vi "test Is OD Entry_3.vi"(11 "Test Case In":refnum<class "test EDS.lvclass">) -> (0 "error out":errorcluster, 3 "Test Case Out":refnum<class "test EDS.lvclass">)   [LabVIEW 2024, in "test EDS.lvclass"]
uses:
  test EDS.lvclass
  C:/Program Files/National Instruments/LabVIEW 2024/vi.lib/Astemes/LUnit/Test Case.lvclass
  <vilib>/Astemes/LUnit/Test Case.lvclass/Test Case.ctl
  b03896ba-5917-454d-83b7-19e02c3a27a5.vi
  <vilib>/Astemes/LUnit/Append Pass Result.vi
  <vilib>/Astemes/LUnit/Append Fail Result.vi
  <vilib>/Astemes/LUnit/Describe Comparison.vi
  b03896ba-5917-454d-83b7-19e02c3a27a5.vi/9c5d11cd-9439-4240-a1ee-d9baace9c924.vi
  <vilib>/Astemes/LUnit/Run In UI.vi
  <vilib>/Utility/error.llb/Clear Errors.vi
  <vilib>/Astemes/LUnit/Describe Variant.vi
  Core/Section Name/Section Name.lvclass
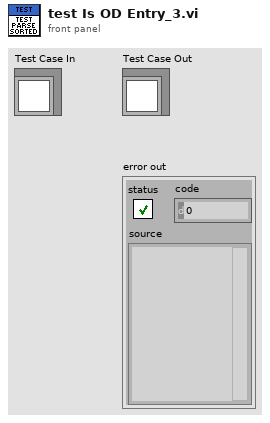
[diagram p1: front panel]
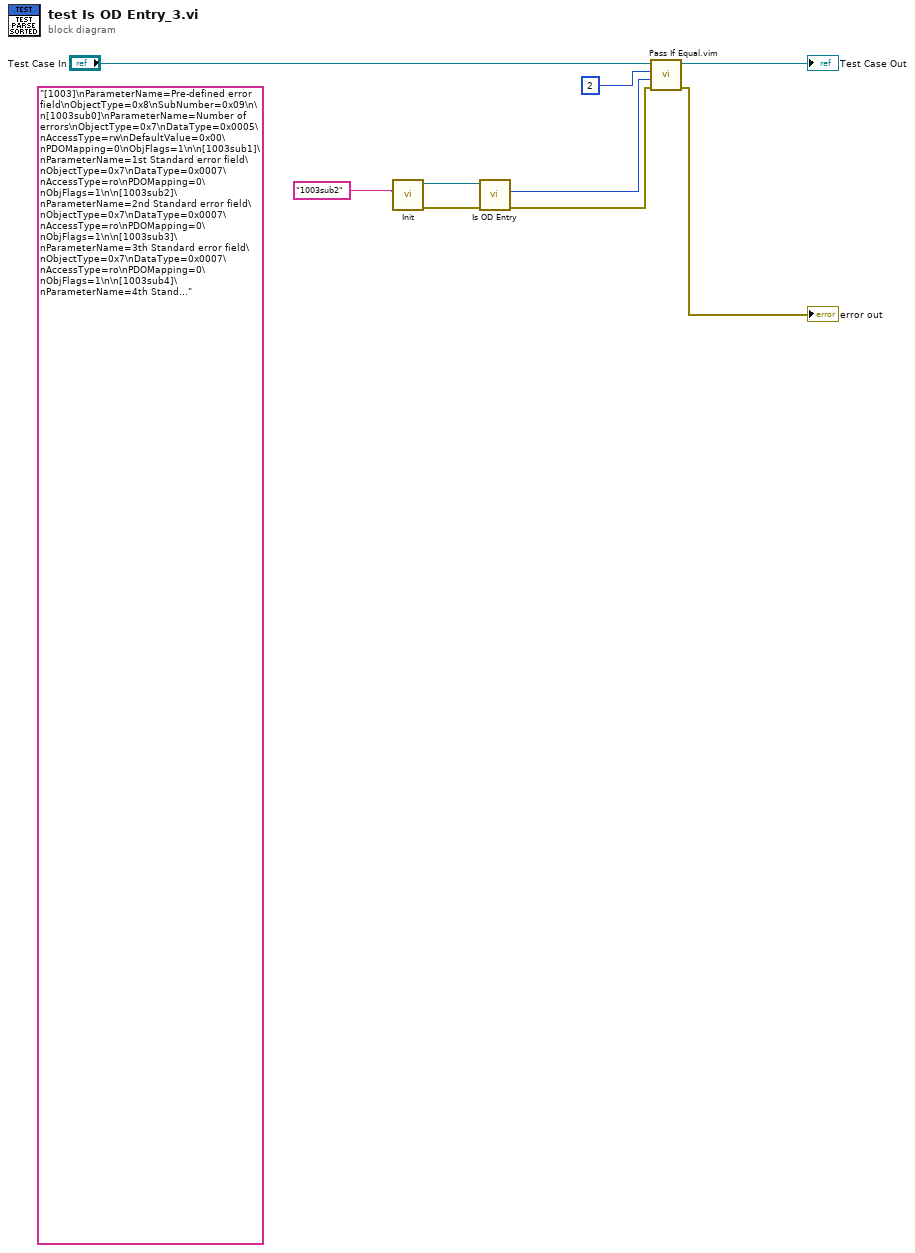
[diagram p0: block diagram]
diagram:
  (unwired) "[1003]\nParameterName=Pre-defined error field\nObjectType=0x8\nSubNumber=0x09\n\n[1003sub0]\nParameterName=Number of errors\nObjectType=0x7\nDataType=0x0005\nAccessType=rw\nDefaultValue=0x00\nPDOMapping=0\nObjFlags=1\n\n[1003sub1]\nParameterName=1st Standard error field\nObjectType=0x7\nDataType=0x0007\nAccessType=ro\nPDOMapping=0\nObjFlags=1\n\n[1003sub2]\nParameterName=2nd Standard error field\nObjectType=0x7\nDataType=0x0007\nAccessType=ro\nPDOMapping=0\nObjFlags=1\n\n[1003sub3]\nParameterName=3th Standard error field\nObjectType=0x7\nDataType=0x0007\nAccessType=ro\nPDOMapping=0\nObjFlags=1\n\n[1003sub4]\nParameterName=4th Standard error field\nObjectType=0x7\nDataType=0x0007\nAccessType=ro\nPDOMapping=0\nObjFlags=1\n\n[1003sub5]\nParameterName=5th Standard error field\nObjectType=0x7\nDataType=0x0007\nAccessType=ro\nPDOMapping=0\nObjFlags=1\n\n[1003sub6]\nParameterName=6th Standard error field\nObjectType=0x7\nDataType=0x0007\nAccessType=ro\nPDOMapping=0\nObjFlags=1\n\n[1003sub7]\nParameterName=7th Standard error field\nObjectType=0x7\nDataType=0x0007\nAccessType=ro\nPDOMapping=0\nObjFlags=1\n\n[1003sub8]\nParameterName=8th Standard error field\nObjectType=0x7\nDataType=0x0007\nAccessType=ro\nPDOMapping=0\nObjFlags=1"
  n1 = call "Init.vi"("Section Name"="1003sub2") -> ("error out"=w5:errorcluster, "Section Name out"=w6:refnum<class "Section Name.lvclass">)  [unwired: 9 in]
  n2 = call "Is OD Entry.vi"("error in"=w5, "Section Name in"=w6) -> ("error out"=w3:errorcluster, "Index"=w2:u16)  [unwired: 6 in, 2 out]
  n3 = call "Pass If Equal.vim"("error in (no error)"=w3, "Actual"=w2, "Expected"=u16 2, "LUnit Test Case In"="Test Case In") -> ("error out"=→"error out":errorcluster, "LUnit Test Case Out"=→"Test Case Out":refnum<class "test EDS.lvclass">)  [unwired: 6 in]
